vi "AddShape Response.vi"(8 "error in (no error)":errorcluster, 9 "Behind":bool, 10 "Shape Reference":refnum<data-value>, 11 "Image Editor Handler in":refnum<class "Image Editor Handler.lvclass">) -> (0 "error out":errorcluster, 3 "Image Editor Handler out":refnum<class "Image Editor Handler.lvclass">)   [LabVIEW 2015, in "LV Image Editor Framework.lvlib" / "Image Editor Handler.lvclass"]
uses:
  Image Editor Handler.lvclass
  Forms/Shape/Shape.lvclass
  Image Editor Handler.lvclass/Image Editor Handler.ctl
  Image/Image.lvclass
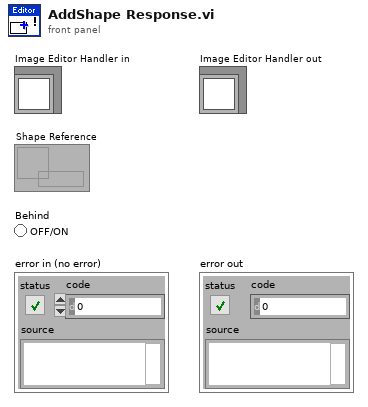
[diagram p1: front panel]
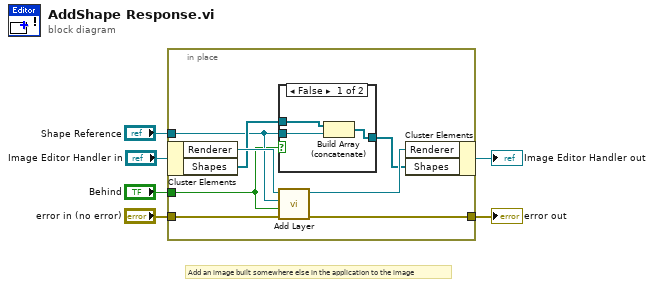
[diagram p0: block diagram]
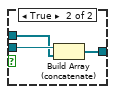
[diagram p2: hidden frame]
diagram:
  # "Add an image built somewhere else in the application to the image"
  n1 = in-place {
    in-place-border: "Shape Reference" -> [w10]
    in-place-border: "Behind" -> [w9]
    in-place-border: [w8] -> w6
    in-place-border: "error in (no error)" -> [w7]
    n2 = in-place-cluster #1("Image Editor Handler in") -> ("Renderer"=w14:refnum<class "Image.lvclass">, "Shapes"=w12:refnum<data-value>[])
    n3 = case shown="False" w9 {
      tunnel: w12 -> [w17 w19]
      tunnel: [w16 w18] -> w11
      tunnel: w10 -> [w15 w20]
      frame False {
        n4 = Build Array (concatenate)(w17, w15) -> (w16:refnum<data-value>[])
      }
      frame True {
        n5 = Build Array (concatenate)(w20, w19) -> (w18:refnum<data-value>[])
      }
    }
    n6 = call "Add Layer.vi"("error in (no error)"=w7, "Behind"=w9, "New ShapeRef"=w10, "Image in"=w14) -> ("error out"=w8:errorcluster, "Image out"=w13:refnum<class "Image.lvclass">)  [unwired: 6 in]
    n7 = in-place-cluster #1("Renderer"=w13, "Shapes"=w11) -> (→"Image Editor Handler out":refnum<class "Image Editor Handler.lvclass">)
  }
  "error out" <- w6
